vi "LS336 Controller_subvi.vi"() -> ()   [LabVIEW 2011]
panel:
  in  "# Steps_Probe":dbl=-1.0
  in  "Stop_Probe":dbl=-60.0 format="%.2f"
  in  "# Step_Rad":dbl=-1.0
  in  "Stop_Rad":dbl=-60.0 format="%.2f"
  out "Remote":bool
  out "Ethernet":bool
  out "Alarm":bool
  out "4":bool
  out "3":bool
  out "2":bool
  out "1":bool
  out "D:  Not Used":dbl
  out "B:  Rad Shield":dbl
  out "C:  Probe Tip":dbl
  out "A:  Sample Stage":dbl
  in  "Sample Control":bool
  out "VISA Resource (TPX)":refnum<visa-resource-name>="GPIB0::12::INSTR"
  in  "Radiation Sheild":bool
  in  "Probe Tip":bool
  in  "Start (K)":dbl format="%.2f"
  in  "# Steps":dbl=-1.0
  in  "Stop (K)":dbl=-60.0 format="%.2f"
  in  "Start Temp (Rad)":dbl format="%.2f"
  in  "Start Temp (Probe)":dbl=-60.0 format="%.2f"
  # "K"
  # "K"
  # "K"
  # "K"
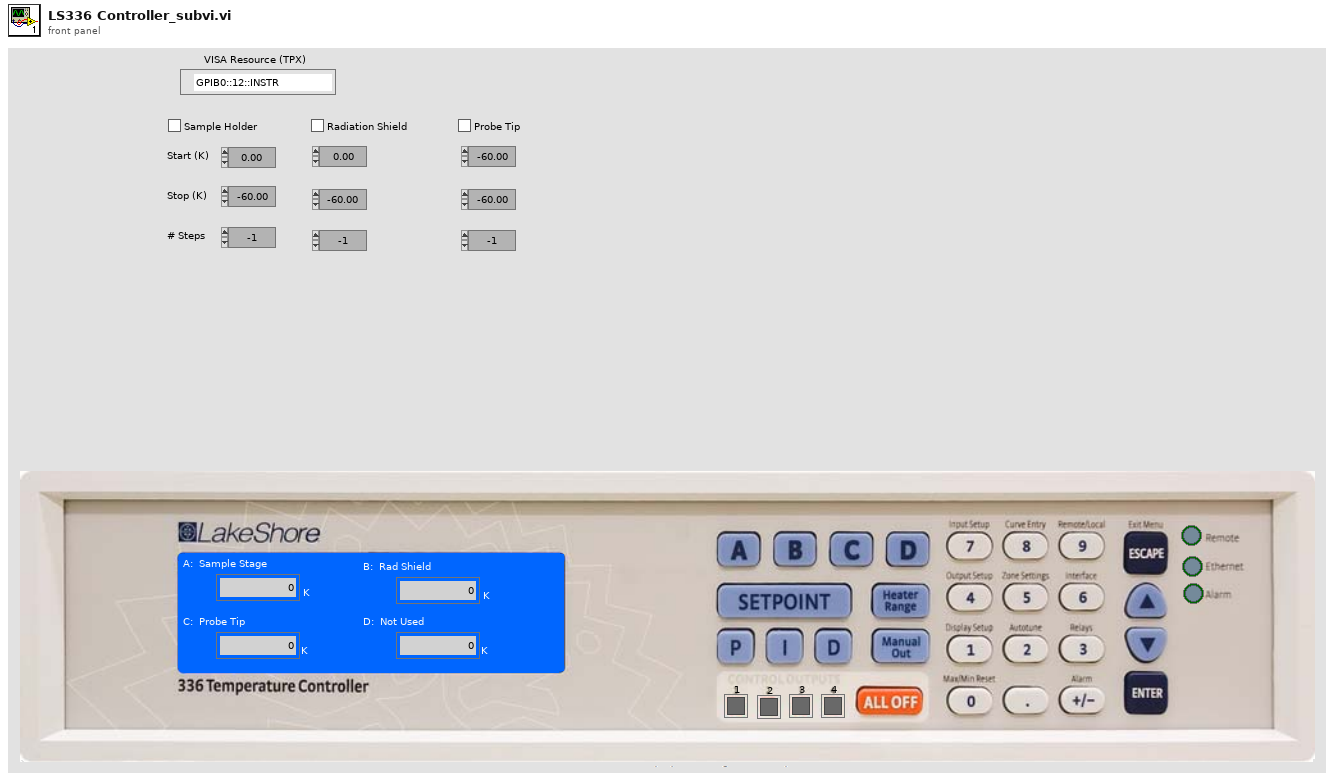
[diagram p1: front panel]
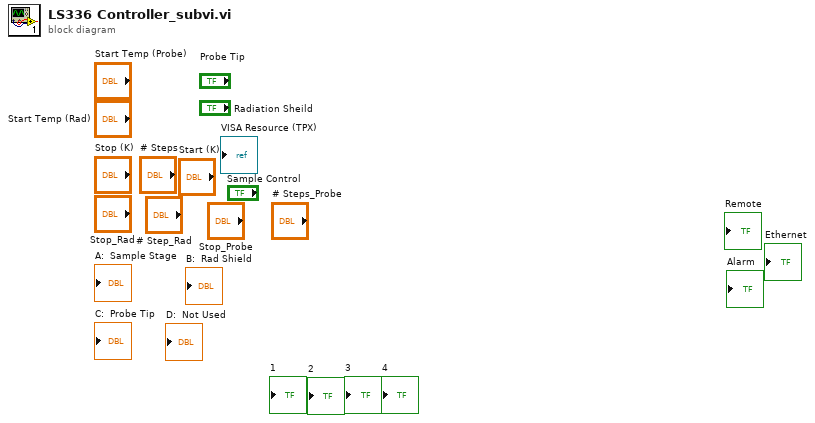
[diagram p0: block diagram]
diagram:
